vi "Drag.vi"(8 "error in (no error)":errorcluster, 9 "delta":cluster{"X":dbl, "Y":dbl}, 11 "FSM in":refnum<class "FSM.Node.lvclass">) -> (0 "error out":errorcluster, 3 "FSM out":refnum<class "FSM.Node.lvclass">)   [LabVIEW 2015, in "FSM.Node.lvclass"]
uses:
  FSM.Node.lvclass
  FSM.Node.lvclass/FSM.Node.ctl
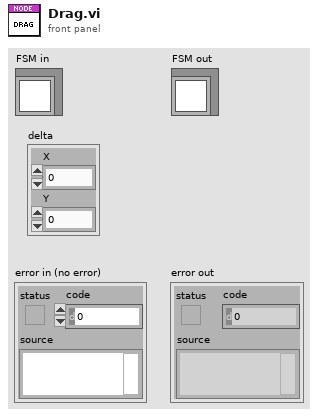
[diagram p1: front panel]
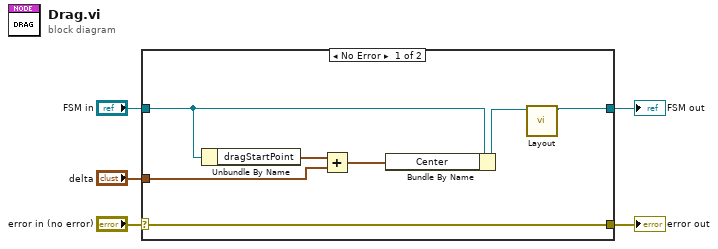
[diagram p0: block diagram]
diagram:
  n1 = case shown="No Error" "error in (no error)" {
    selector: "error in (no error)" -> [w12 w14]
    tunnel: [w12 w14] -> w4
    tunnel: [w8 w13] -> w2
    tunnel: "FSM in" -> [w7 w13]
    tunnel: "delta" -> [w6 _]
    frame No Error {
      n2 = Unbundle By Name(w7) -> ("dragStartPoint"=w11:cluster{"x":i16, "y":i16})
      n3 = Add(x=w11, y=w6) -> (x+y=w10:cluster{dbl, dbl})
      n4 = Bundle By Name(cluster=w7, "Center"=w10) -> (w9:refnum<class "FSM.Node.lvclass">)
      n5 = call "Layout.vi"("FSM in"=w9) -> ("FSM out"=w8:refnum<class "FSM.Node.lvclass">)  [unwired: 9 in, 1 out]
    }
    frame Error {
    }
  }
  "error out" <- w4
  "FSM out" <- w2
